vi "Initialize.vi"(8 "error in (no error)":errorcluster, 10 "Properties String":string, 11 "CSSProperties in":refnum<class "CSSProperties.lvclass">) -> (0 "error out":errorcluster, 3 "CSSProperties out":refnum<class "CSSProperties.lvclass">)   [LabVIEW 2019, in "CSSProperties.lvclass"]
uses:
  CSSProperties.lvclass
  CSSProperties.lvclass/CSSProperties.ctl
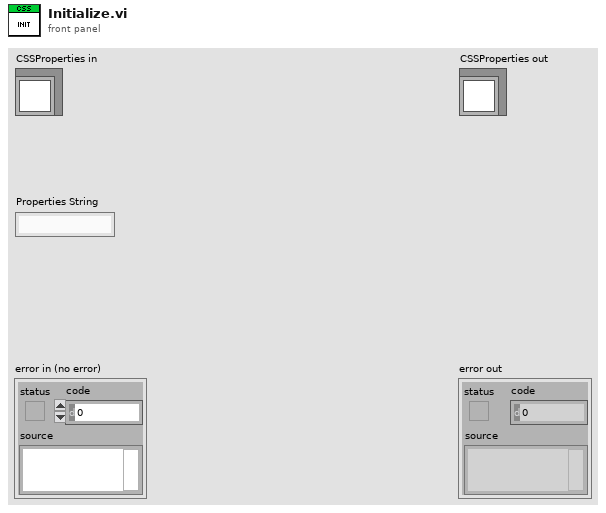
[diagram p1: front panel]
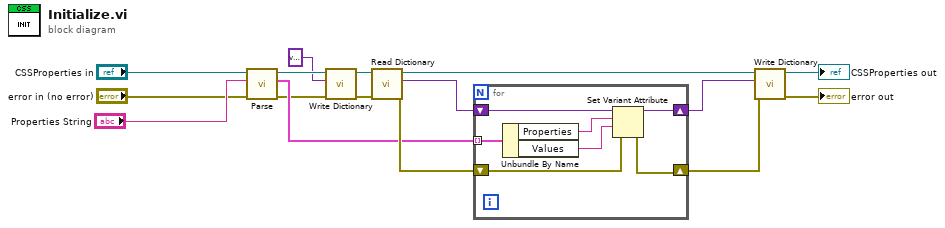
[diagram p0: block diagram]
diagram:
  n1 = call "Parse.vi"("error in (no error)"="error in (no error)", "Properties String"="Properties String", "CSSProperties in"="CSSProperties in") -> ("error out"=w2:errorcluster, "KVPs"=w6:cluster{"Properties":string, "Values":string}[], "CSSProperties out"=w5:refnum<class "CSSProperties.lvclass">)  [unwired: 6 in]
  n2 = call "Write Dictionary.vi"("error in (no error)"=w2, "Dictionary"=variant, "CSSProperties in"=w5) -> ("error out"=w1:errorcluster, "CSSProperties out"=w4:refnum<class "CSSProperties.lvclass">)  [unwired: 7 in]
  n3 = call "Read Dictionary.vi"("error in (no error)"=w1, "CSSProperties in"=w4) -> ("error out"=w9:errorcluster, "Dictionary"=w8:variant, "CSSProperties out"=w13:refnum<class "CSSProperties.lvclass">)  [unwired: 7 in]
  n4 = for {
    tunnel: w6 -> [w23] mode=indexing
    shift-right: [w21] -> w7
    shift-left: w8 -> [w22]
    shift-right: [w17] -> w11
    shift-left: w9 -> [w18]
    n5 = Unbundle By Name(w23) -> ("Properties"=w20:string, "Values"=w19:string)
    n6 = Set Variant Attribute(Variant=w22, name=w20, value=w19, error in=w18) -> (Variant out=w21:variant, error out=w17:errorcluster)  [unwired: 1 out]
  }
  n7 = call "Write Dictionary.vi"("error in (no error)"=w11, "Dictionary"=w7, "CSSProperties in"=w13) -> ("error out"=→"error out":errorcluster, "CSSProperties out"=→"CSSProperties out":refnum<class "CSSProperties.lvclass">)  [unwired: 7 in]
